vi "StopConnectionManager.vi"(0 "STOMP in":refnum<class "STOMP.lvclass">, 5 "error in (no error)":errorcluster) -> (14 "STOMP out":refnum<class "STOMP.lvclass">, 16 "stop?":bool, 19 "error out":errorcluster)   [LabVIEW 2017, in "STOMP.lvclass"]
uses:
  STOMP.lvclass
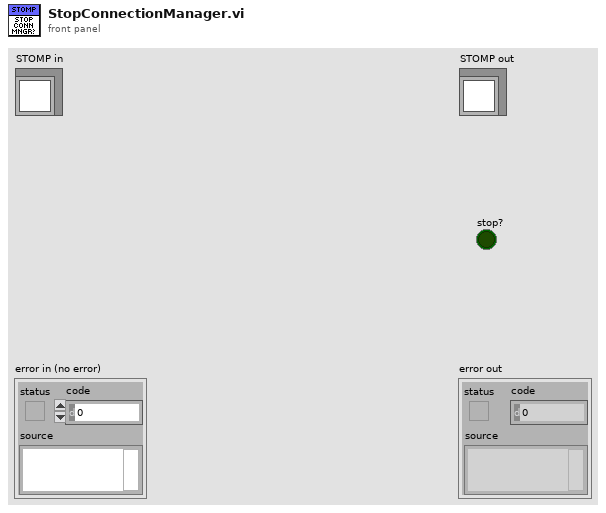
[diagram p1: front panel]
types:
  T1 = typedef "STOMP.lvclass/ObjectAttributes.ctl" = cluster{"address":string, "port":u16, "ConnectionRef":refnum<k5>, "messageQueue":refnum<queue>, "receiptQueue":refnum<queue>, "errorQueue":refnum<queue>, "sendQueue":refnum<queue>, "currentReceiptNumber":u64, "currentSubscriptionId":u64, "closeConnection":bool, "activeSubscriptions":T2[]}
  T2 = typedef "STOMP.lvclass/Type_ActiveSubscription.ctl" = cluster{"id":u64, "receipt":bool, "Destination":string, "ack":T3, "headers":T4[]}
  T3 = typedef "STOMP.lvclass/Type_AckHeader.ctl" = enum16{"auto", "client", "client-individual"}
  T4 = typedef "STOMP.lvclass/Type_FrameHeader.ctl" = cluster{"Header":string, "Value":string}
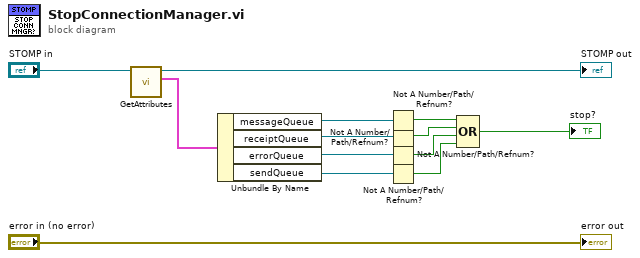
[diagram p0: block diagram]
diagram:
  n1 = call-dynamic "GetAttributes.vi"("STOMP in"="STOMP in") -> ("attributes"=w5:T1, "STOMP out"=→"STOMP out":refnum<class "STOMP.lvclass">)  [unwired: 8 in, 1 out]
  n2 = Unbundle By Name(w5) -> ("messageQueue"=w12:refnum<queue>, "receiptQueue"=w10:refnum<queue>, "errorQueue"=w11:refnum<queue>, "sendQueue"=w2:refnum<queue>)
  n3 = Not A Number/Path/Refnum?(number/path/refnum=w12) -> (NaN/Path/Refnum?=w9:bool)
  n4 = Not A Number/Path/Refnum?(number/path/refnum=w10) -> (NaN/Path/Refnum?=w8:bool)
  n5 = Not A Number/Path/Refnum?(number/path/refnum=w11) -> (NaN/Path/Refnum?=w7:bool)
  n6 = Not A Number/Path/Refnum?(number/path/refnum=w2) -> (NaN/Path/Refnum?=w1:bool)
  n7 = Compound Arithmetic op=OR(w9, w8, w7, w1) -> (→"stop?":bool)
  "error out" <- "error in (no error)"
